vi "OUTPUT_BP4610.vi"(8 "error in":errorcluster, 10 "Output":bool, 11 "port in":refnum<visa-resource-name> caption="VISAsession") -> (0 "error out":errorcluster, 3 "port out":refnum<visa-resource-name> caption="CopyVISAsession")   [LabVIEW 2019]
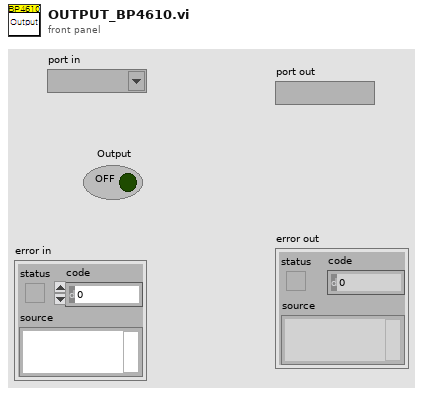
[diagram p1: front panel]
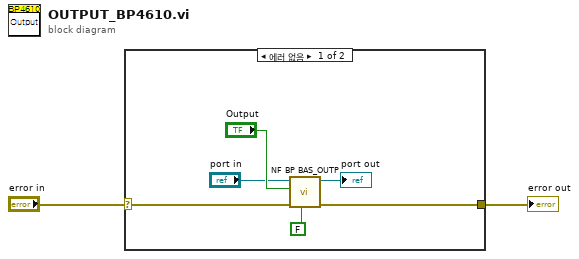
[diagram p0: block diagram]
diagram:
  n1 = case shown="에러 없음" "error in" {
    selector: "error in" -> [w6 w9]
    tunnel: [w5 w9] -> w1
    frame No Error {
      n2 = call <instrlib>:"NF BP BAS_OUTP.vi"("Read(F)"=FALSE ("Read"), "error in (no error)"=w6, "State(OFF)"="Output", "VISAsession"="port in") -> ("error out"=w5:errorcluster, "CopyVISAsession"=→"port out":refnum<visa-resource-name>)  [unwired: 4 in, 2 out]
    }
    frame Error {
    }
  }
  "error out" <- w1
